vi "2023_day14.vi"() -> ()   [LabVIEW 2021]
uses:
  39e69416-e89b-4aea-9585-c6c336cbe10e.vi
  <userlib>/_OpenG.lib/array/array.llb/Search 1D Array (String)__ogtk.vi
  <userlib>/_OpenG.lib/array/array.llb/Remove Duplicates from 1D Array (I32)__ogtk.vi
  <userlib>/_OpenG.lib/array/array.llb/Sort 1D Array (I32)__ogtk.vi
  <userlib>/_OpenG.lib/array/array.llb/Search 1D Array (I32)__ogtk.vi
  <userlib>/_OpenG.lib/array/array.llb/Sort 2D Array (I32)__ogtk.vi
  <vilib>/Comparison/Less/Less Functor/Less Functor.lvclass
panel:
  out "Table Control":string[][](table)
  out "Task 1":i32
  out "Task 2 - Middle point guess":i32
  in  "Switch":bool caption="Ex. Data  vs.  User Data"
  # "Task 2 - brute force estimate"
  # "TIP: Try Middle point value first and then try moddle of the next interval where it throws you. Good luck with guessing ..."
  # "64 - match (test data)\n90551 - match (live data)"
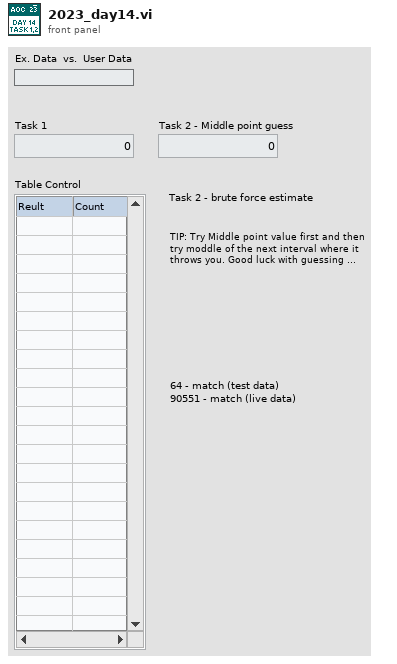
[diagram p1: front panel]
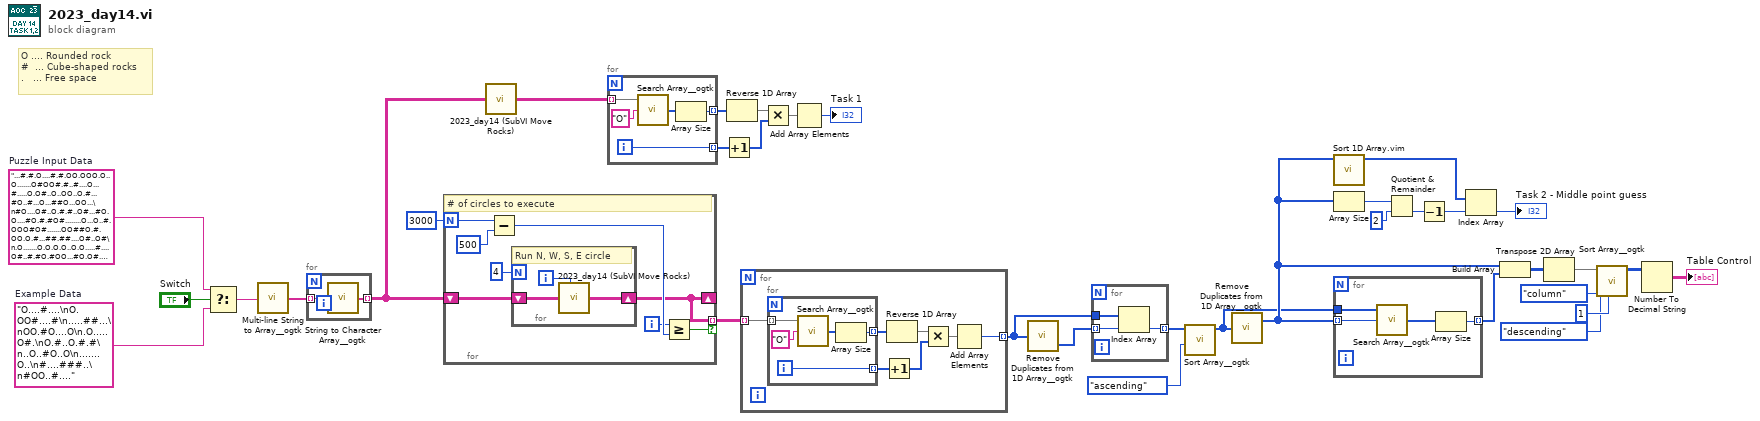
[diagram p0: block diagram]
diagram:
  w33 = "...#.#.O....#.#.OO.OOO.O..O.......O#OO#.#..#....O...#.....O.O#..O..OO..O.#...#O..#...O...##O...OO...\n#O....O#..O.#.#..O#...#O.O....#O.#.#O#........O...O..#.OOO#O#.......OO##O.#.OO.O.#...##.##....O#..O#\n.O.......O.O.O.O..O.O.....#....O#..#.#O.#OO...#O.O#.O#..#O...#...O.O.......#.O....O.#..#.O##O#..O...\n...O....#.OO..#..OO#..##....#O.......OOOOOO...OO..#...#.O..O....#O..OO.#O...#O#...O..O#..OO....#....\n..O...##OOO....#..OO.OO#O##..#.#........O#.#.....#OO...#............#.###..#.#O...#..O.#O#.O#O.....#\n...............O.....##..O...O#.O#........#.O.#..#...#..O..O.#...#......#......O.OO.OOO.#.O.....O##.\n......#..#..###.OO.#......O..O.O##O..O.....OO.#.OO....O.....OO#O..O....#.....#.#.O#..O..O.OO.O#O.O.#\n##O.....O.#.#O...#.#O###....#.O#.#..#..O.#O........O.OO..#..#O#.O#..OO..#.O.##O....#.##O.O.......##.\nO#...###...O..#...#......O#.OO.....#...OOO...#.#O.#...##..OO#.......#OO.....#...O...#.#O.........O.O\n..O....O....OO..O.O.O........#.O#..O.#..#..OO#.OO..#.O...O..#...O..##..O........O##..........OOO..OO\n....##......#.#.O.O#O##.#....#..O#............#..#...#......#O.OO#....O.......O###....O...........OO\n.O.OOO..O#....O...O..#.O#.#O.O...#.O..O#...OO#.#....#OO.#........#O.......O...#O......O...O....#...#\n.#....#O...##..#.#..........O..#O........OOO.......O.OO.##...#..........#......#.O##.#O#OO#OO..#..O.\n......#O...#.#.......O........#O....#O..##....O......O.#.O..#OO............O##O....#O.OO#..O#..O#...\n..OO.....O#O..#OOOO#O.##.........O..#OO#......O.OO.....O......OO..O...O..O....O..O#O.......O..O.O#..\n....O...OO....##.....OOO...O#O.#.O...O.....#........#.#O#.....O.O.OO.###.#.OO#OO....O.....O..#.#O...\n.OO#..O#O#O...#..O.O....O#.O.#........O.O..O....#O#....#.#.O#.#...O.O..O..#..#...OO#O......#O.O..O.#\nOO...O.O.#..#....#...#O.O##O#...#............##.O..OOO....O..OO....#OO....O.#....O#.O........OO..#..\n..O#.OO#.#O#..O.......O.##.O.#....OO#.#O#.##.O..O#..####....#..#......#...##.O##...O....O..#.#......\n#O.O#.....#....O...O.O..O.O.O#O.O#....#..O...#.O.#O...#..#.#O.....#O..##...O.......O.....O..OO#OO##.\n..O.#..#...O....#.##.#.O......#.#.##.......#.O..##O#.#O.OOO..O...#O......#..O.....O.OO...O#.O.#OO#.O\n.#..OO#.......OO....O.##...O......O.OO#.O......#O..O#..#..O.O..O.#..OO.O.#O..O..#......O...O....O#..\nO....#.#O..O#...#..##..##.O.O.O..O.O#...O#..#O.O......#O.......O..O.O...#.#O..OO#.#.....#O#...O..#.O\n...O...O.O.O.OO..O....O..O..O##..O.........O#O..O.#...#.O..O.#........#...O........O#.#.O..O.....#..\nOO....O#...........#OO......O.....O...#...OO....OO..O.........O.#......##O....#...O##....O.#...#...#\n#OO#....#......OO.O....O...#..O...#.OOOO..OOO.O.O...O#.......O....#O#O.O#O......#...#...OO#.O...#..#\n....O#.#...O..#.................#.#...O...O...O.O#.##..O.#.#....####..OO....O.......#.OO.O....#...#.\n.....O.#.#O..#O...#OO....OO...O#..O...O..#O..O....#.#O..#.......O...O.O.....#.##.#O.OO..#.#....###..\n.#O..#...#...#.#.O.#O.#OO..#.#..#O#.#.#O#.O#O#..##..#...#O#.#..#.OO#..#..#..O...O...O..O...#.O....O.\n..O.....#....#O#OO#O.....O.....O...OO.O......OO..O....O...#....O....#...OO....O..O...#...###O.....#.\n##..##...#OOO...#.OO...#.#.O#.O.........O.O.#.O..O.OO#.O......#.###...#..#O.#....#...#.O..##...#O...\n.O.#...O.O....O.......O...#O.....O......OO..OOO##.#...##OO.O......#....O..#..#.##.OO.......#O...#OO.\n...#...O#..O.#.OO.#.OO..O.#O.#.O.#...O#....O#.O#......OO.#....#..#..#..#....O.#....##...............\n.O.O#....#.#.....O...#.O#O#.......#.#O..OO.O...#....#.....O.#.#.#..#...#...##..O.O...#O..O.#..#O....\n.#......O..O#...O.O.##O..#.OOOO.O#O....O#...#O..OO.#.#O......#..O..O.OO#OOO#O#.O.......OO.....O...#O\nO##.O..OOO.#..O......#...#O#.O.O#..O.OO..#......O.O.O..O.O.OO..#....O.#O...O#.#..#..O.#...##O.O.....\n.#OO#....#.....#..OO.OO...##.O......OOO.#O..O#.O.O.........O#.O.#.#...#..##...#O.O..OO.O#.#..O..O.O.\n.O.....#.O#....O#.....#.O..O..O#..#..OOO#O....#OOOOO.#.#.........O#..O.#....#.#....O.#..##..#.......\n..O.#OO....#O.#...#O...#.O#..#.O....O.#..O....O#.....O.OO..OO.OO#.#..#..#O.O.#...O....OO...O.#..O..O\n.O.OO#...O#.OO....#.O....O.###...#..O.....O....#.O..O.#O.O.....#....#O#O...#..O...O........O...#....\n#...#...#..O..#.##.#.....O#..#O.##.O...O...#....O.O.O..O.O........O.O.O.....O..#.......#...O..O.#.#O\n#O...#...O.#....#.O.....OOO..O...OO#OO#.......#O.##...#.O#O#....#.....O#..OO.#.#.O.O..O.#OO.O.#..O..\n......O.......O.#.O.#.O...........O.O.OO#....#OO........O#.......OO.O..#O...#....O#..O....OO..O##...\n.##..O..#O...O.O....#O#..OO#O.#....#O.OO#O....#.....#...#.#OO#.OO.#.O.O.O.OO.#O.O.#.O....#O.O.O..O..\nO#..O#O##.O....O..#......O....#..O##O.O#...O...O...OO#..#OO...O##.#....O#.O..O.......#..#......#O..#\nO.OO..O..#.O..O#OO#O.....#O..O..#...#.OO.O..O...........O...O...OO##.#..O..#.#.OO.#.#...O.O......O.O\n.O.O##.O....#O.O...O#.#..O....#O.....O..O#OO....OO##.#.O..#O.O...O..O.O...#O.OO.........#.##OO#..#..\n..OO....O.....#....O.....O...OOO#...#.O.........O.O..OOO.###O.#.......#.#...O.OO.#..O.....#O.....#..\nO...##O...O..##..#.#...#.#O#.O...#.#.O..O....##......#...#.O..O...OO.#...OOO#OO...O.O#O..OO.O##O..O.\n..#.OO.#.##..O....#...OO.#O.......O.O#...O..#.#O..O.###O#.#.O.O...O.#O.#..#.O..O#O#..O.........#.#..\nO.#.O##.......OO#....O#.......O..O.....#.........O.O.....#O.......#O..#.O...#....O.#....#......O.O.#\n.OO.O...O.......#O#....#O#...#.........O..O.#.OO#.OO.O#...#O...O..#..O##O.#...O#..O.OO.O...#OO.##.#.\n...O.O...OOO.O......#..O...#.##.O..O..#...O.O...#.O.O..OO..OO..#....O.O#..#...O.OO.#.....#...OO#...#\n.#............#O.OO..O#.....O..#O.#O.##O....O.O....O..O#..O..O.#..O.#.O.#.O.#..#O.#.OO.O......##...O\n#.....O.#..O.O........O#O#OO..OO.....#.#....OO##......O.O.##..##.#.O...O.#.#O......O..##.#.#.#..#O..\n##.#.O..O...O..OO...O....O.O..O#...OO....OO#.#...#.#....OO#..........O..O...O...O........#..O##.#.#.\n..OO.#..#.OO..#O..#.O...OO.O...O....#..OO....#OO..#........#...O..........#..O...OO.O.......#.#..##.\n.#.#...#O.O.#.O..O.OO.OO#..OO#OOO#O....O..O#..OO.O..##..#.#....OOOOO#....OO..O....#..O..............\n...O#.OO......O.#.O.#.#O.OOO...#OO..#....#.O.O.O.......#...##...O...OOO..##...O....O...O.#...O.O...O\n..O...O..#.O.....#.#..##.......####...##.......O...O#.##....O.#..OO....#.#.O...##O.#O.###.OO#....O.O\n.O#..#....OO...O.O.......O#OO..O#.O.O..#......#..O.#..#O......OO.O...O.....O........O#.#O.#.#.##.O#.\n..O....O.#...#..##..O...#.O#..OO...O.......#OOO......#O..OO...O...#..O...##O.#...#.#.##...O...#.OO..\nO.#..#...O#OO.O#.O..O.....O.O..#.#.##....O.O..O......OO.O.#.....#....#.##...#...O..O........#......#\n.OO.OO.........#...#.#O...#..#..#.###O....#...OO#......#O.O..........#O...#.#.#O#..........#.O#...OO\n##.#..#O#OO.#.....O......#....O..#.O#..#.OO.........#.......#.#..#..O.O#OO.###.O.#.#O..##....O.O..O#\n#...O...O.......O#.O.#..#O#.O...O...O...O.O.#.O....O###..#.O..O.....O..OO#...O.#...#....O.#O..OO.O..\n#O...O...O.##..#.#OO.....#O.#..O....#O.O....O.....#.O.....#.O.O....#.......O.#.O..#.O.##....O..O..O#\nO..O.....#O..O...O........O..#.#..........##O#..#..O.#.#OOO..#..O...O..O..#.O....O...O...#...#...O..\n#...O.......O#..#.O#.O.....#....O#O......O..O.....#.....O...#...O...#O..#.O..#..#....O....##O#.....#\nO...O..#O#.OO..##..#.......O.........#......#...#..O.O..#..#O..O..O.OO......O#OO.#..O#....#.O.#.....\n.....#.OOO..OOO....O...#O....O.#.O.#.#O..#O.......O#..O.#O.#.#..#......O#O###..#.#.O..OO.O#.##.OO#.#\nO...#..O#.##O..#...#.....O...O.O............O#.....#.O....O#....O#.#O#O..O#.OO..........#.O.#OOO.O..\n......#..#...O..O....OO#.O...OO..O....O..##O#..O#..O..##.O..#....##OO.....#..O#.O....#O.#....##.O...\n.#..O.O..#..........O...O...O.#..O.#......O.O.....OO#..#...O.....O##..O.O..#.OO.#O.O....O...O..#..#.\n.OO.#..O......#........#.#.O...#..........O..O.O.......OO..##O.....#...O...#..#O###..O..O.OOOOO.#.O.\n.O..#..O..O...O..#O......OOO.O#..O#.#O...O#O.#...O....O..OO.#....#...O#................O.#O..O.#O..#\n......O..O...##..O..##.O.####..OO.O.......#.#O..O#..O#O.......#..O.....##........#..O..O.#...O....OO\n.....O.O.O.....O..OO..#O..O#.#OO....#O...#O#.#.OO.#..O...O.#.....#.#O#..O#...OO##.........##...##..#\n....O..OOOO..O.O...#.....#.#..OOO...#OO.O#..O..O....#O.......#.O..OOO......OO...#.O#............O#.O\n......O....#...#.#..O.O#.#...O..O.OO##.O..O#OO##...#.#..O.OO.........#..##O#...O.#..O.#OO.#O#...##O.\nO..##.O...O..#.O.O.O..O.........#..O...#..O.O.##O#.O..#.#.....#..#O#..#.OOO#.O..O...OO#.O...O#......\n.O.....O......O.......O#..O.OOOO..O..OO.O#.##.OO#O#.O......#...#.........O..O#...#O..#..#.O...O.#OO.\n#O.O...#..OO.#...O.O#....#..#...#OOO##.O.OO#.....#.O#.O..O.#O#O.O.O..........O#.O#.#O###O..#..#.#OO#\n#O###.O..O..O......#.O#.#....OO..O.O#....#...#...#.##...OO..O.#OO........O....O..O....OO......O..O.#\n.O#O..O...#OOO...O.O...#.O#......#......#O.....O.#.#.O.#....O#.#O..#...#..#...OO#.....OOO....OO.....\n..O.#.O....OO......O...O..##.O........#.O.#O.#...O...O.#.##OO.#O......O...O..O.O.O.##..O#.##.#.#O...\n.#OO#.#.O#O....O.O....OO#....##.....#.##O..O...OO.....#..O.#....O#.......O....OO.OOO.#...#..O.O.#.OO\n.O...O....#.O..O.#..#.........O.#O#.#...O..#O.O.O..O##.....OO..O.O..OO..O..#..#.#.O..#O..O.OO##....O\n.##...#O.O..OO..O..#.#O.O.OO.#..#.OOOO.....O...O.O.O#...O#.#.O.............O..O...#.#..........OO#.#\n.#....##O....##O..#.O.O..#..O##....#.#.OO........O.O#..#........#OO........O...#.OO..#.........#....\n.##OO..#O.#.O..OO.#...#O#.....O....O.#....#O..O#O.#.O..##.O.O.....#.#...#.O..OO....O....#.#.#.......\nO.O.O.#....#.OO.#...#...O..#.OO..#..O..#...O.OO.O...##...OO.O#O..O.OO.O##.....#..O#..#O....O.O#OO.#.\n.#.O....#.#....#..O.O....OO......O......O.#...O...#.O.O..#.#.....O..#O.O.O..OOO#.O#..O...O#..OO.....\n#.#O..#....#.....O.#....#......O.O..O.O.OO.O#...O.#.O.O...#....O...#..#...O.#.O..#.O...OO.#.#O###.OO\n..#..O..#O##..#.....O...#..O...OO..#.#.O.#.O.O.....O..O#O#..O......#...#O.O.OO..O............#....#.\n....O#....O#O###O.O..#.#..O.#.O.#.O....O........#O.OOO......O.OO....O.O.O.....##.O#....##O.#.OO..O.#\n..#.O...OO.#O.#..OO.##..#...O#..O#..#O.O..#......O.....##....O...O.O#OO#O.......O##OOO.OO.O...O.#..#\nO......#.O.....OO.OO.O...O.#O..O...O.#.#...#...O...#.OO.O.#.#OO.....#.O.#....OOO........##...##.##O.\n#O...#....#...##O.#......O#...#O..........##O..#.O.#O#..#...OO.O....O..##..#...#...#..O..O....O..O#.\n...OO....O#..O..#....O.#.#.....OO.#..#O..OO.#.#.#.#......O...O..#.#..##.....#...O.##.....O#.#..O#O.."  # Puzzle Input Data
  w34 = "O....#....\nO.OO#....#\n.....##...\nOO.#O....O\n.O.....O#.\nO.#..O.#.#\n..O..#O..O\n.......O..\n#....###..\n#OO..#...."  # Example Data
  # "O .... Rounded rock\n#  ... Cube-shaped rocks \n.   ... Free space"
  n1 = Select(t=w33, s="Switch", f=w34) -> (s? t:f=w32:string)
  n2 = call <userlib>:"Multi-line String to Array__ogtk.vi"("string"=w32) -> ("lines"=w31:string[])
  n3 = for {
    tunnel: w31 -> [w37] mode=indexing
    tunnel: [w36] -> w23 mode=indexing
    n4 = call <userlib>:"String to Character Array__ogtk.vi"("Input String"=w37) -> ("Character Array"=w36:string[])
  }
  n5 = for {
    N: 3000 -> [w43]
    shift-right: [w39] -> _
    shift-left: w23 -> [w45]
    tunnel: [w39] -> w21 mode=indexing if=w38
    i -> [w40]
    # "# of circles to execute"
    n6 = Subtract(x=w43, y=500) -> (x-y=w41:i32)
    n7 = for {
      N: 4 -> [_]
      shift-right: [w46] -> w39
      shift-left: w45 -> [w47]
      i -> [w48]
      # "Run N, W, S, E circle"
      n8 = call "2023_day14 (SubVI Move Rocks).vi"("Roll Direction"=w48, "Map In"=w47) -> ("Map Out"=w46:string[][])  [unwired: 7 in]
    }
    n9 = Greater Or Equal?(x=w40, y=w41) -> (x >= y?=w38:bool)
  }
  n10 = call "2023_day14 (SubVI Move Rocks).vi"("Map In"=w23) -> ("Map Out"=w24:string[][])  [unwired: 8 in]
  n11 = for {
    tunnel: w24 -> [w51] mode=indexing
    tunnel: [w50] -> w27 mode=indexing
    tunnel: [w49] -> w30 mode=indexing
    i -> [w49]
    n12 = call-poly <userlib>:"Search Array__ogtk.vi"("Array"=w51, "Element Data"="O") -> ("Indices of Elements"=w53:i32[])  [unwired: 7 in]
    n13 = Array Size(array=w53) -> (size(s)=w50:i32)
  }
  n14 = Increment(x=w30) -> (x+1=w25:i32[])
  n15 = Reverse 1D Array(array=w27) -> (reversed array=w29:i32[])
  n16 = for {
    tunnel: w21 -> [w55] mode=indexing
    tunnel: [w54] -> w19 mode=indexing
    n17 = for {
      tunnel: [w63] -> w58 mode=indexing
      tunnel: [w62] -> w56 mode=indexing
      tunnel: w55 -> [w61] mode=indexing
      i -> [w62]
      n18 = call-poly <userlib>:"Search Array__ogtk.vi"("Array"=w61, "Element Data"="O") -> ("Indices of Elements"=w65:i32[])  [unwired: 7 in]
      n19 = Array Size(array=w65) -> (size(s)=w63:i32)
    }
    n20 = Increment(x=w56) -> (x+1=w60:i32[])
    n21 = Reverse 1D Array(array=w58) -> (reversed array=w57:i32[])
    n22 = Multiply(x=w57, y=w60) -> (x*y=w59:i32[])
    n23 = Add Array Elements(numeric array=w59) -> (sum=w54:i32)
  }
  n24 = Multiply(x=w29, y=w25) -> (x*y=w26:i32[])
  n25 = Add Array Elements(numeric array=w26) -> (sum=→"Task 1":i32)
  n26 = call-poly <userlib>:"Remove Duplicates from 1D Array__ogtk.vi"("Input Array"=w19) -> ("indices of removed elements"=w20:i32[])  [unwired: 1 out]
  n27 = for {
    tunnel: w20 -> [w68] mode=indexing
    tunnel: w19 -> [w67]
    tunnel: [w66] -> w18 mode=indexing
    n28 = Index Array(array=w67, index=w68) -> (element=w66:i32)
  }
  n29 = call-poly <userlib>:"Sort Array__ogtk.vi"("Order"=enum16{"ascending", "descending"}."ascending", "Array in"=w18) -> ("Sorted Array out"=w1:i32[])  [unwired: 8 in, 1 out]
  n30 = call-poly <userlib>:"Remove Duplicates from 1D Array__ogtk.vi"("Input Array"=w1) -> ("Output Array"=w10:i32[])  [unwired: 1 out]
  n31 = call "Sort 1D Array.vim"("unsorted array"=w10) -> ("sorted array"=w6:i32[])  [unwired: 10 in]
  n32 = Array Size(array=w10) -> (size(s)=w9:i32)
  n33 = for {
    tunnel: w10 -> [w70] mode=indexing
    tunnel: w1 -> [w72]
    tunnel: [w69] -> w16 mode=indexing
    n34 = call-poly <userlib>:"Search Array__ogtk.vi"("Array"=w72, "Element Data"=w70) -> ("Indices of Elements"=w71:i32[])  [unwired: 7 in]
    n35 = Array Size(array=w71) -> (size(s)=w69:i32)
  }
  n36 = Quotient & Remainder(x=w9, y=2) -> (floor(x/y)=w7:i32)  [unwired: 1 out]
  n37 = Decrement(x=w7) -> (x-1=w5:i32)
  n38 = Index Array(array=w6, index=w5) -> (element=→"Task 2 - Middle point guess":i32)
  n39 = Build Array(w10, w16) -> (w15:i32[][])
  n40 = Transpose 2D Array(2D array=w15) -> (transposed array=w11:i32[][])
  n41 = call-poly <userlib>:"Sort Array__ogtk.vi"("Column/Row to Sort By"=u32 1, "Sort By in"=enum16{"row", "column"}."column", "Order"=enum16{"ascending", "descending"}."descending", "Array in"=w11) -> ("Sorted Array out"=w4:i32[][])  [unwired: 4 in, 3 out]
  n42 = Number To Decimal String(number=w4) -> (decimal integer string=→"Table Control":string[][])  [unwired: 1 in]
